vi "ClearBranchName.vi"(11 "Node In":refnum<data-value>) -> (2 "Node Name Out":string, 3 "Node Out":refnum<data-value>)   [LabVIEW 2019]
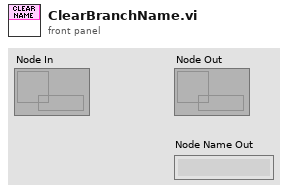
[diagram p1: front panel]
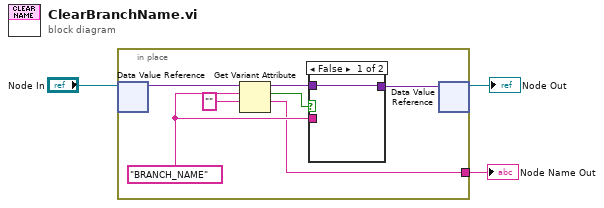
[diagram p0: block diagram]
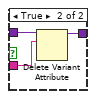
[diagram p2: hidden frame]
diagram:
  n1 = in-place {
    in-place-border: [w5] -> w1
    w6 = "BRANCH_NAME" ("Unique Node Name")
    n2 = in-place-dvr #1("Node In") -> (w9:variant)  [unwired: 1 out]
    n3 = Get Variant Attribute(Variant=w9, name=w6, default value (empty Variant)="") -> (duplicate Variant=w8:variant, found=w4:bool, value=w5:string)  [unwired: 1 in, 1 out]
    n4 = case shown="False" w4 {
      tunnel: [w11 w14] -> w10
      tunnel: w8 -> [w11 w13]
      tunnel: w6 -> [_ w12]
      frame False {
      }
      frame True {
        n5 = Delete Variant Attribute(6:w12, 7:w13) -> (3:w14:variant)  [unwired: 1 in, 2 out]
      }
    }
    n6 = in-place-dvr #1(w10) -> (→"Node Out":refnum<data-value>)  [unwired: 1 out]
  }
  "Node Name Out" <- w1
